vi "Tx.vi"(8 "error in (no error)":errorcluster, 10 "Command Parameters":T1, 11 "Dispatcher in":refnum<class "Dispatcher Thread.lvclass">) -> (0 "error out":errorcluster, 3 "Dispatcher out":refnum<class "Dispatcher Thread.lvclass">)   [LabVIEW 2017, in "DSF Core.lvlib" / "Dispatcher Thread.lvclass"]
uses:
  Dispatcher Thread.lvclass
  Interfaces/Dispatcher/Parameters.ctl
  Interfaces/Dispatcher/Tx Parameters.ctl
  Interfaces/Plugin/Command.ctl
  Dispatcher Thread.lvclass/Dispatcher Thread.ctl
  Thread Pool/Plugin Interface Pool.lvclass/Plugin Interface Pool.ctl
  Thread Pool/Pool.lvclass/Pool.ctl
  Interfaces/Interface/Interface.lvclass/Interface.ctl
  Thread Pool/Read FIFO.vi
  Interfaces/Plugin/Send.vi
  Interfaces/Plugin/Send Plugin Command.vi
  Interfaces/Interface/Send Command.vi
  Interfaces/Interface/Write RT FIFO.vi
  Thread Pool/Plugin Interface Pool.lvclass
  C:/Git/DSF/Data Sharing Framework Core/Classes/Thread Pool/Pool.lvclass
  Interfaces/Plugin/Plugin Interface.lvclass
  C:/Git/DSF/Data Sharing Framework Core/Classes/Interfaces/Interface/Interface.lvclass
  Interfaces/Plugin/Class Name.vi
  VIs/VI Name.vi
  Interfaces/Interface/Errors.vi
  Interfaces/Dispatcher/Command Timeout.vi
  Interfaces/Dispatcher/Dispatcher Interface.lvclass
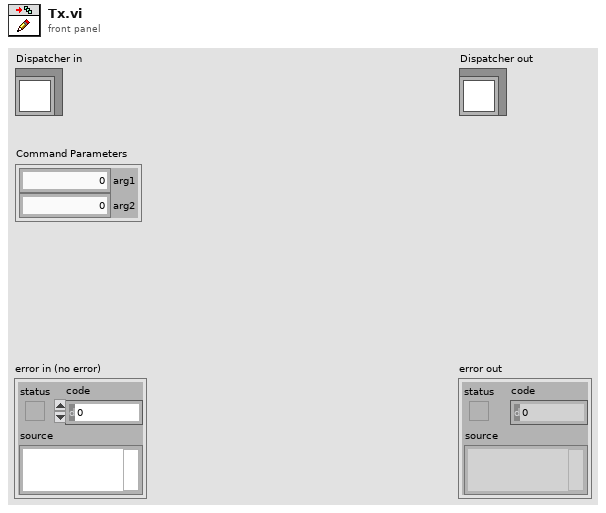
[diagram p1: front panel]
types:
  T1 = typedef "DSF Core.lvlib/Dispatcher Interface.lvclass/Parameters.ctl" = cluster{"arg1":u64, "arg2":u64}
  T2 = typedef "DSF Core.lvlib/Plugin Interface.lvclass/Command.ctl" = enum8{"Set Inline Buffer", "Rx", "Tx", "Shutdown"}
  T3 = typedef "DSF Core.lvlib/Dispatcher Interface.lvclass/Tx Parameters.ctl" = cluster{"Plugin ID":i32, "Transfer Group ID":i32, "Iteration":u64}
  T4 = typedef "DSF Core.lvlib/Dispatcher Thread.lvclass/Plugin Settings.ctl" = cluster{"Transfer Group threads":i32[], "Plugin Thread Pool":refnum<class "Plugin Interface Pool.lvclass">}
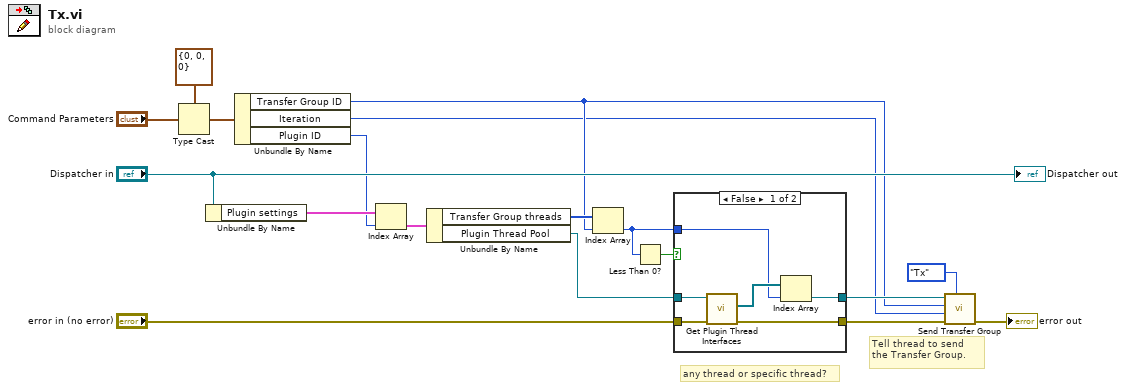
[diagram p0: block diagram]
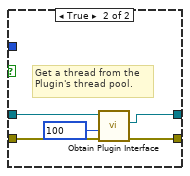
[diagram p2: hidden frame]
diagram:
  # "any thread or specific thread?"
  # "Tell thread to send the Transfer Group."
  n1 = Type Cast(type=T3 {"Plugin ID"=0, "Transfer Group ID"=0, "Iteration"=0}, x="Command Parameters") -> (*(type *) &x=w16:T3)
  n2 = Unbundle By Name("Dispatcher in") -> ("Plugin settings"=w15:T4[])
  n3 = Unbundle By Name(w16) -> ("Transfer Group ID"=w2:i32, "Iteration"=w1:u64, "Plugin ID"=w13:i32)
  n4 = Index Array(array=w15, index=w13) -> (element=w10:T4)
  n5 = Unbundle By Name(w10) -> ("Transfer Group threads"=w9:i32[], "Plugin Thread Pool"=w5:refnum<class "Plugin Interface Pool.lvclass">)
  n6 = Index Array(array=w9, index=w2) -> (element=w6:i32)
  n7 = Less Than 0?(x=w6) -> (x < 0?=w7:bool)
  n8 = case shown="False" w7 {
    tunnel: "error in (no error)" -> [w19 w26]
    tunnel: w6 -> [w20 _]
    tunnel: w5 -> [w23 w27]
    tunnel: [w21 w25] -> w4
    tunnel: [w19 w24] -> w3
    frame False {
      n9 = call "Get Plugin Thread Interfaces.vi"("Plugin Interface Pool in"=w23) -> ("Plugin Thread Interfaces"=w22:refnum<class "Plugin Interface.lvclass">[])  [unwired: 9 in, 1 out]
      n10 = Index Array(array=w22, index=w20) -> (element=w21:refnum<class "Plugin Interface.lvclass">)
    }
    frame True {
      # "Get a thread from the Plugin's thread pool."
      n11 = call "Obtain Plugin Interface.vi"("error in (no error)"=w26, "timeout in ms (0)"=100, "Plugin Interface Pool in"=w27) -> ("error out"=w24:errorcluster, "Plugin Interface"=w25:refnum<class "Plugin Interface.lvclass">)  [unwired: 5 in, 2 out]
    }
  }
  n12 = call "Send Transfer Group.vi"("Command"=Command."Tx", "error in (no error)"=w3, "Transfer Group iteration"=w1, "Transfer Group ID"=w2, "Plugin Interface in"=w4) -> ("error out"=→"error out":errorcluster)  [unwired: 5 in, 1 out]
  "Dispatcher out" <- "Dispatcher in"
